vi "Open Command.vi"   [LabVIEW 2015, in "SLSC Interfaces.lvlib" / "SLSC Interface.lvclass"]
uses:
  SLSC Interface.lvclass
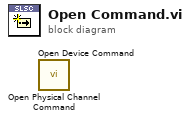
[diagram p0: block diagram]
diagram:
  n1 = call "Open Physical Channel Command.vi"() -> ()  [unwired: 13 in, 3 out]
  n2 = call "Open Device Command.vi"() -> ()  [unwired: 13 in, 3 out]
